vi "Display UI.vi"(8 "error in (no error)":errorcluster, 11 "Configuration in":refnum<class "Configuration.lvclass">) -> (0 "error out":errorcluster, 3 "Configuration out":refnum<class "Configuration.lvclass">)   [LabVIEW 2026, in "Configuration.lvlib" / "Configuration.lvclass"]
doc: "This method displays the actor core of the leaf in the class hierarchy. This ensures that only the most specific definition of a UI is displayed, and no ancestors are seen by the user"
uses:
  Configuration.lvclass
  Configuration.lvclass/Configuration.ctl
  Accessors/Write VI to Display.vi
  Accessors/Read VI to Display.vi
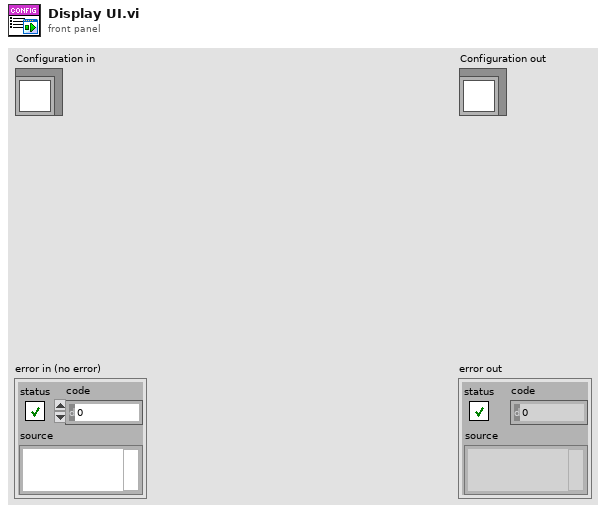
[diagram p1: front panel]
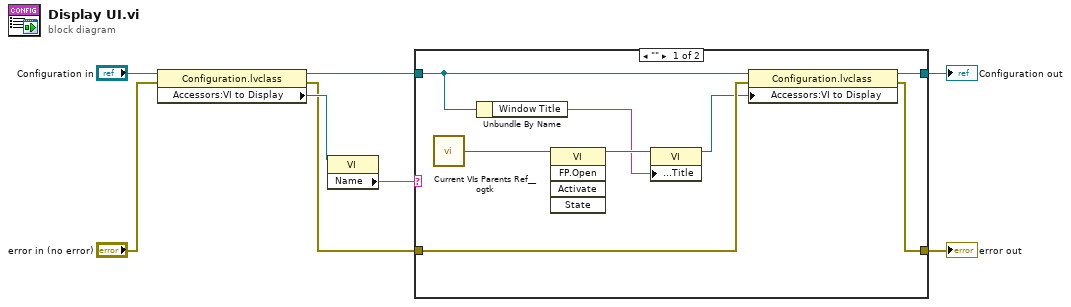
[diagram p0: block diagram]
diagram:
  n1 = property class="Configuration.lvclass"(reference="Configuration in", error in="error in (no error)") -> (reference out=w6:refnum<class "Configuration.lvclass">, error out=w2:errorcluster, "Accessors:VI to Display"=w5:refnum<vi>)
  n2 = property class="VI"(reference=w5) -> ("Name"=w4:string)  [unwired: 1 in, 2 out]
  n3 = case shown="\"\"" w4 {
    tunnel: [w15 w18] -> w7
    tunnel: w6 -> [w10 w18]
    tunnel: w2 -> [w13 w17]
    tunnel: [w12 w17] -> w1
    frame "" {
      n4 = call <userlib>:"Current VIs Parents Ref__ogtk.vi"() -> ("Calling VI's Reference"=w16:refnum<vi>)  [unwired: 2 in]
      n5 = Unbundle By Name(w10) -> ("Window Title"=w9:string)
      n6 = invoke class="VI" method="FP.Open"(reference=w16) -> (reference out=w14:refnum<vi>)  [unwired: 4 in, 4 out]
      n7 = property class="VI"(reference=w14, "Front Panel.Title"=w9) -> (reference out=w11:refnum<vi>)  [unwired: 1 in, 1 out]
      n8 = property class="Configuration.lvclass"(reference=w10, error in=w13, "Accessors:VI to Display"=w11) -> (reference out=w15:refnum<class "Configuration.lvclass">, error out=w12:errorcluster)
    }
    frame Default {
    }
  }
  "error out" <- w1
  "Configuration out" <- w7
